vi "Check restric Dryness Load Size.vi"(8 "Error In":errorcluster, 10 "All_ERD_Data_Bundled_Brass out":T2, 11 "Read ERD List":T1[](array[typedef]) {"ERD Number" format="%.0x"}) -> (0 "Error Out":errorcluster, 2 "New ERD Data":T1[](array[typedef]) {"ERD Number" format="%.0x"})   [LabVIEW 2023]
uses:
  type defs/All_Bundled_Data_JL.ctl
  Common/type defs/Version.ctl
  type defs/ERD_Always_Show_JL.ctl
  Common/type defs/CSV_File_String_Arrays.ctl
  Common/type defs/Fault Table Array.ctl
  Common/type defs/Fault_Table_Info.ctl
  type defs/Heat Control.ctl
  type defs/ERD_Commercial_Laundry.ctl
  Common/type defs/BootloaderVersion.ctl
  type defs/ERD_RJ45.ctl
  Common/LabVIEW GEA2 Toolkit/GEA3/type defs/ERD Read Data In.ctl
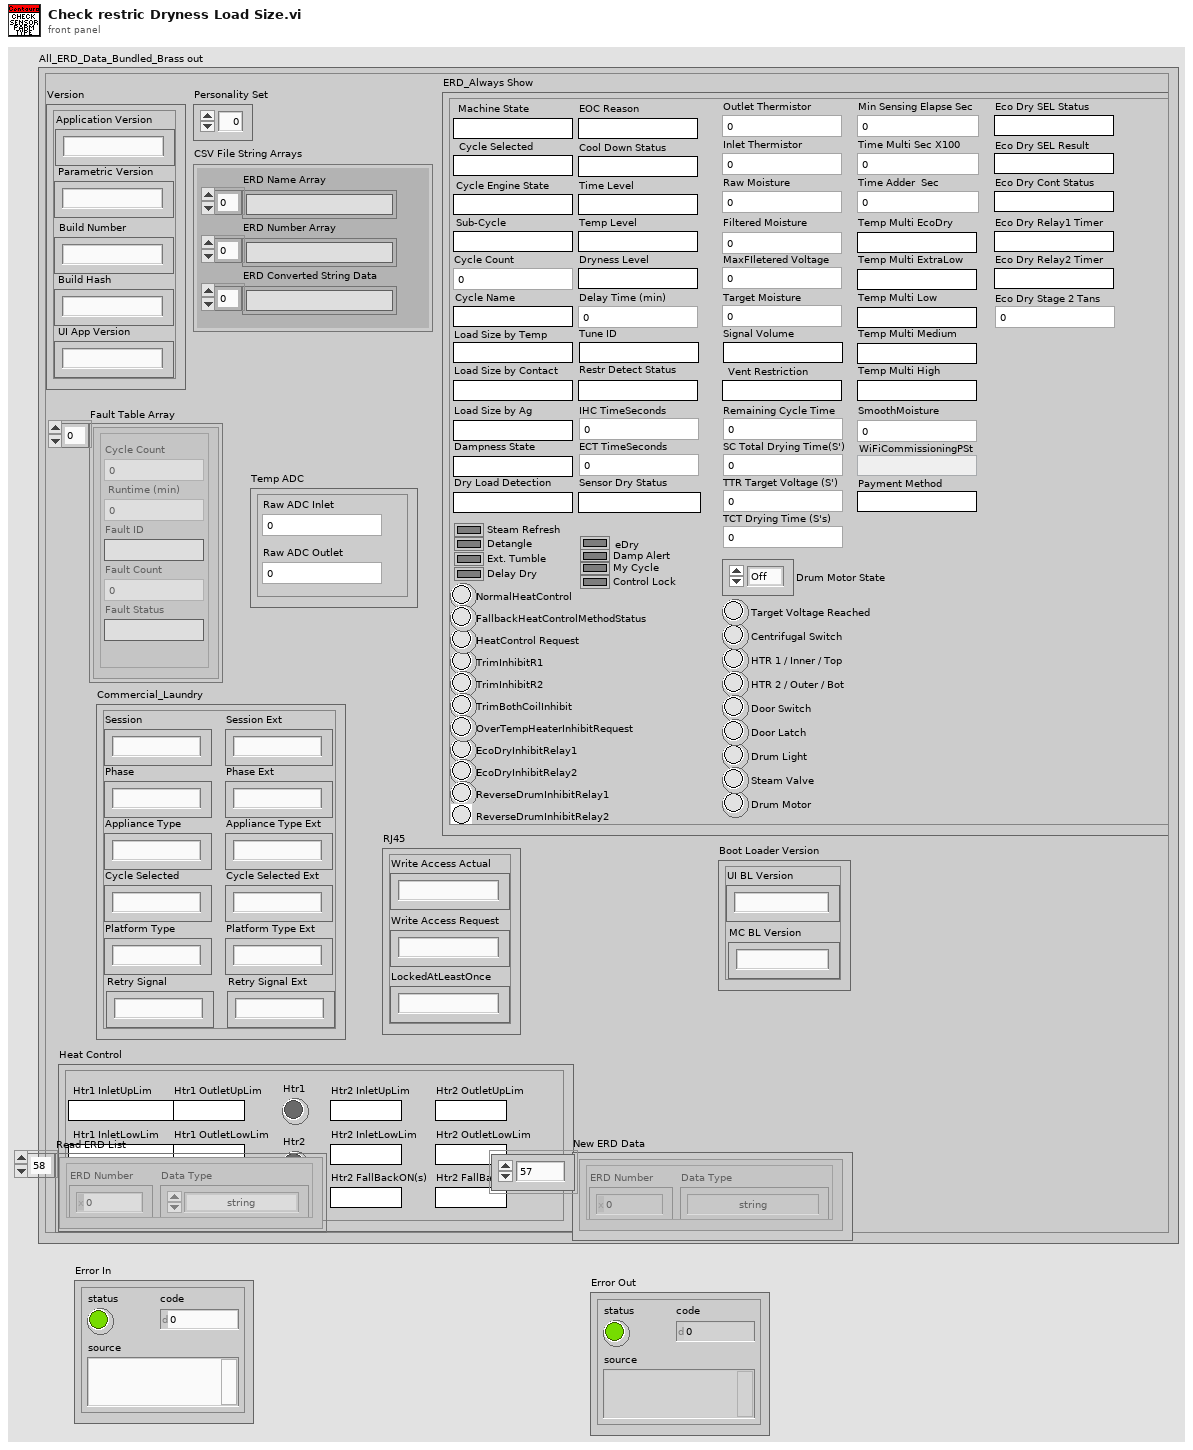
[diagram p1: front panel]
types:
  T1 = typedef "ERD Read Data In.ctl" = cluster{"ERD Number":u16, "Data Type":enum16{"string", "boolean", "uint8_t", "uint16_t", "uint32_t", "uint64_t", "int8_t", "int16_t", "int32_t", "int64_t"}}
  T2 = typedef "All_Bundled_Data_JL.ctl" = cluster{"Version":T3, "ERD_Always Show":T4, "Personality Set":u8, "CSV File String Arrays":T5, "Fault Table Array ":T6, "Heat Control":T8, "Temp ADC":cluster{"Raw ADC Outlet":u16, "Raw ADC Inlet":u16}, "Commercial_Laundry":T9, "Boot Loader Version":T10, "RJ45":T11}
  T3 = typedef "Version.ctl" = cluster{"Build Number":string, "Build Hash ":string, "Application Version":string, "Parametric Version":string, "UI App Version":string}
  T4 = typedef "ERD_Always_Show_JL.ctl" = cluster{"Inlet Thermistor":u16, "Machine State":string, "Filtered Moisture":u16, "Cycle Selected":string, "HTR 1 / Inner / Top":bool, "HTR 2 / Outer / Bot":bool, "Door Switch":bool, "Drum Light":bool, "Cycle Engine State":string, "Centrifugal Switch":bool, "Drum Motor":bool, "Cycle Count":u32, "Ext. Tumble":bool, "eDry":bool, "Temp Level":string, "Dryness Level":string, "Time Level":string, "Delay Time (min)":u16, "Steam Refresh":bool, "Damp Alert":bool, "Sub-Cycle":string, "Outlet Thermistor":u16, "Target Moisture":u16, "Remaining Cycle Time":u32, "Raw Moisture":u16, "Cycle Name":string, "My Cycle":bool, "Delay Dry":bool, "Detangle":bool, "Control Lock":bool, "Steam Valve":bool, "Door Latch":bool, "Signal Volume":string, "Tune ID":string, "Restr Detect Status":string, "Vent Restriction":string, "Load Size by Contact":string, "Load Size by Temp":string, "EOC Reason":string, "Sensor Dry Status":string, "Dampness State":string, "Target Voltage Reached":bool, "TrimInhibitR1":bool, "TrimInhibitR2":bool, "TrimBothCoilInhibit":bool, "NormalHeatControl":bool, "HeatControl Request":bool, "Cool Down Status":string, "EcoDryInhibitRelay1":bool, "EcoDryInhibitRelay2":bool, "ReverseDrumInhibitRelay1":bool, "ReverseDrumInhibitRelay2":bool, "OverTempHeaterInhibitRequest":bool, "FallbackHeatControlMethodStatus":bool, "IHC TimeSeconds":u32, "ECT TimeSeconds ":u32, "SC Total Drying Time(S')":u32, "TTR Target Voltage (S')":u32, "TCT Drying Time (S's)":u32, "Drum Motor State":enum16{"Off", "Cw", "Ccw", "Max"}, "Load Size by Ag":string, "MaxFIletered Voltage":u16, "Dry Load Detection":string, "Min Sensing Elapse Sec":u32, "Time Multi Sec X100":u32, "Time Adder  Sec":u32, "Temp Multi EcoDry":string, "Temp Multi ExtraLow":string, "Temp Multi Low ":string, "Temp Multi Medium":string, "Temp Multi High":string, "SmoothMoisture":u16, "Eco Dry SEL Status":string, "Eco Dry SEL Result":string, "Eco Dry Cont Status":string, "Eco Dry Relay1 Timer":string, "Eco Dry Relay2 Timer ":string, "Eco Dry Stage 2 Tans ":u32, "WiFiCommissioningPSt":string, "Payment Method":string}
  T5 = typedef "CSV_File_String_Arrays.ctl" = cluster{"ERD Number Array":string[], "ERD Name Array":string[], "ERD Converted String Data":string[]}
  T6 = typedef "Fault Table Array.ctl" = T7[]
  T7 = typedef "Fault_Table_Info.ctl" = cluster{"Cycle Count":u32, " Runtime (min) ":u32, "Fault Status":string, "Fault ID":string, "Fault Count":u16}
  T8 = typedef "Heat Control.ctl" = cluster{"Htr1 InletLowLim":string, "Htr1 InletUpLim":string, "Htr1 OutletLowLim":string, "Htr1 OutletUpLim":string, "Htr1 FallBackON(s)":string, "Htr1 FallBackOFF(s)":string, "Htr1":bool, "Htr2 InletLowLim":string, "Htr2 InletUpLim":string, "Htr2 OutletLowLim":string, "Htr2 OutletUpLim":string, "Htr2 FallBackON(s)":string, "Htr2 FallBackOFF(s)":string, "Htr2":bool}
  T9 = typedef "ERD_Commercial_Laundry.ctl" = cluster{"Session":string, "Phase":string, "Appliance Type":string, "Cycle Selected":string, "Platform Type":string, "Retry Signal":string, "Session Ext":string, "Phase Ext":string, "Appliance Type Ext":string, "Cycle Selected Ext":string, "Platform Type Ext":string, "Retry Signal Ext":string}
  T10 = typedef "BootloaderVersion.ctl" = cluster{"UI BL Version":string, "MC BL Version":string}
  T11 = typedef "ERD_RJ45.ctl" = cluster{"Write Access Actual":string, "Write Access Request":string, "LockedAtLeastOnce":string}
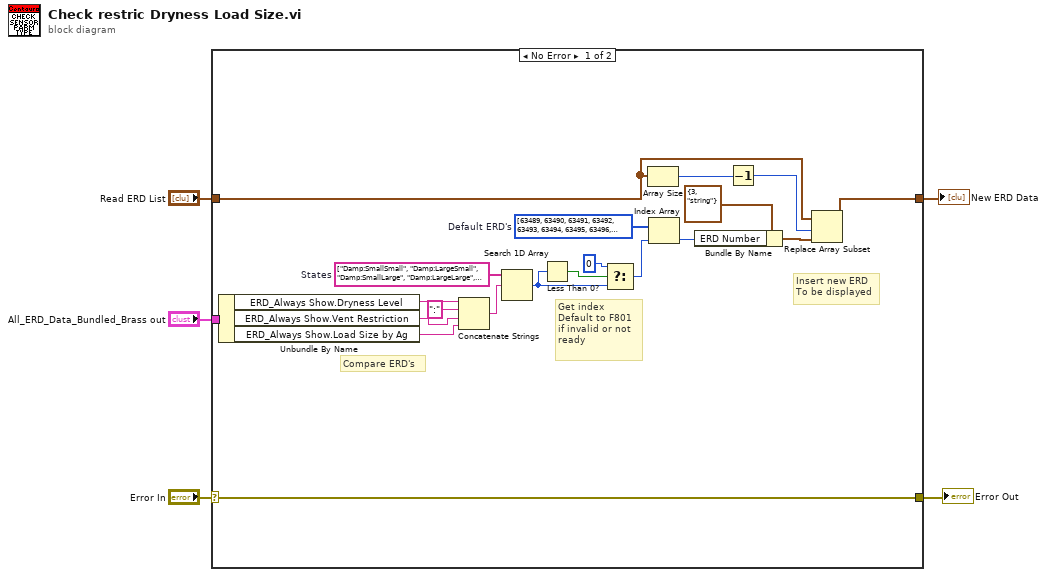
[diagram p0: block diagram]
diagram:
  n1 = case shown="No Error" "Error In" {
    selector: "Error In" -> [w6 w26]
    tunnel: "All_ERD_Data_Bundled_Brass out" -> [w9 _]
    tunnel: "Read ERD List" -> [w8 w27]
    tunnel: [w7 w27] -> w2
    tunnel: [w6 w26] -> w1
    frame No Error {
      w20 = u16[] [63489, 63490, 63491, 63492, 63493, 63494, 63495, 63496, 63497, 63498, 63499, 63500, 63501, 63502, 63503, 63504, 63505, 63506, 63507, 63508]  # Default ERD's
      w22 = string[] ["Damp:SmallSmall", "Damp:LargeSmall", "Damp:SmallLarge", "Damp:LargeLarge", "Less Dry:SmallSmall", "Less Dry:LargeSmall", "Less Dry:SmallLarge", "Less Dry:LargeLarge", "Dry:SmallSmall", "Dry:LargeSmall", "Dry:SmallLarge", "Dry:LargeLarge", "More Dry:SmallSmall", "More Dry:LargeSmall", "More Dry:SmallLarge", "More Dry:LargeLarge", "Extra Dry:SmallSmall", "Extra Dry:LargeSmall", "Extra Dry:SmallLarge", "Extra Dry:LargeLarge"]  # States
      # "Insert new ERD \nTo be displayed"
      # "Get index\nDefault to F801\nif invalid or not \nready"
      # "Compare ERD's"
      n2 = Unbundle By Name(w9) -> ("ERD_Always Show.Dryness Level"=w15:string, "ERD_Always Show.Vent Restriction"=w25:string, "ERD_Always Show.Load Size by Ag"=w21:string)
      n3 = Concatenate Strings(w15, ":", w25, w21) -> (w23:string)
      n4 = Search 1D Array(1D array=w22, element=w23) -> (index of element=w16:i32)  [unwired: 1 in]
      n5 = Less Than 0?(x=w16) -> (x < 0?=w19:bool)
      n6 = Select(t=0 ("index of element"), s=w19, f=w16) -> (s? t:f=w17:i32)
      n7 = Array Size(array=w8) -> (size(s)=w11:i32)
      n8 = Index Array(array=w20, index=w17) -> (element=w13:u16)
      n9 = Bundle By Name(cluster=T1 {"ERD Number"=3, "Data Type"=enum."string"} ("ERD Read Data In"), "ERD Number"=w13) -> (w12:T1)
      n10 = Decrement(x=w11) -> (x-1=w10:i32)
      n11 = Replace Array Subset(array=w8, new element=w12, index=w10) -> (w7:T1[])
    }
    frame Error {
    }
  }
  "Error Out" <- w1
  "New ERD Data" <- w2
